vi "CLD 12 CSV file commands utility.vi"(8 "Error In":errorcluster) -> (0 "Error Out":errorcluster, 3 "Command Array Out":T1[](array[typedef]))   [LabVIEW 2019]
doc: "CLD 12: File access utility. This VI converts the text command to the enum equivalent."
uses:
  CLD 12 Data Cluster.ctl
  CLD 12 Sequencer Enum.ctl
  <vilib>/Utility/file.llb/Read Delimited Spreadsheet (string).vi
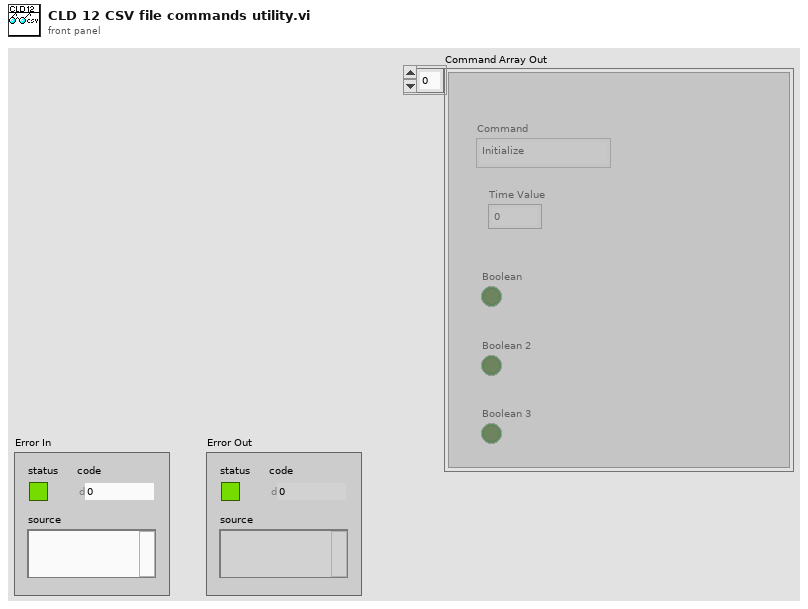
[diagram p1: front panel]
types:
  T1 = typedef "CLD 12 Data Cluster.ctl" = cluster{"Command":T2, "Time Value":dbl, "Boolean":bool, "Boolean 2":bool, "Boolean 3":bool}
  T2 = typedef "CLD 12 Sequencer Enum.ctl" = enum16{"Initialize", "SetTime", "RunState1", "Runstate2", "Idle", "Start"}
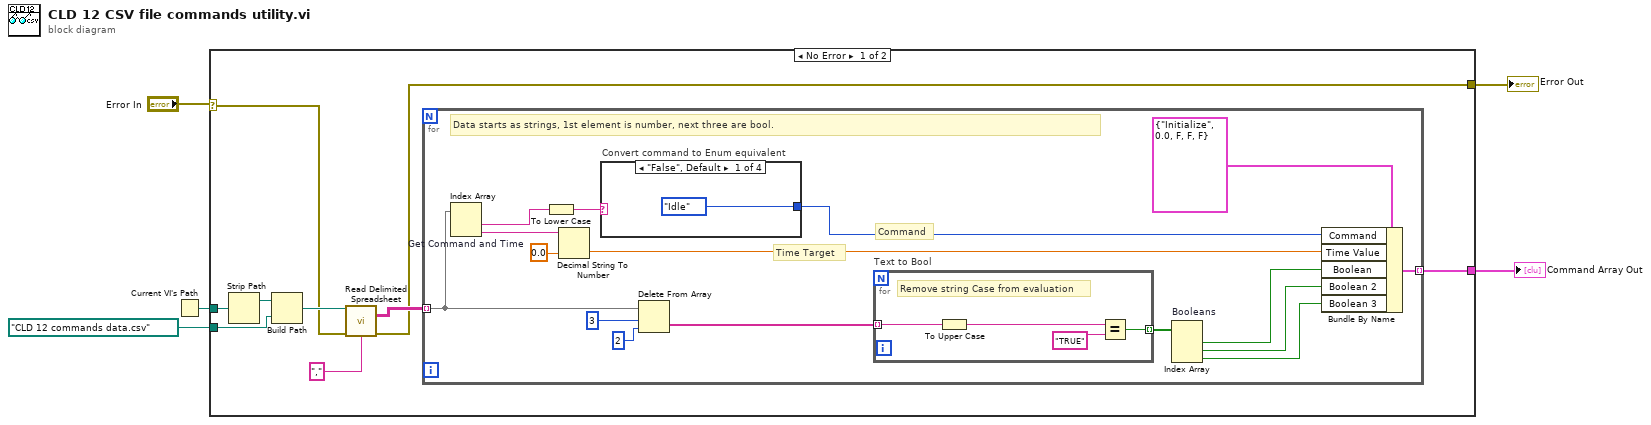
[diagram p0: block diagram]
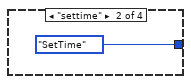
[diagram p2: hidden frame]
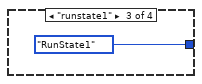
[diagram p3: hidden frame]
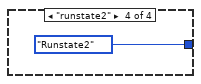
[diagram p4: hidden frame]
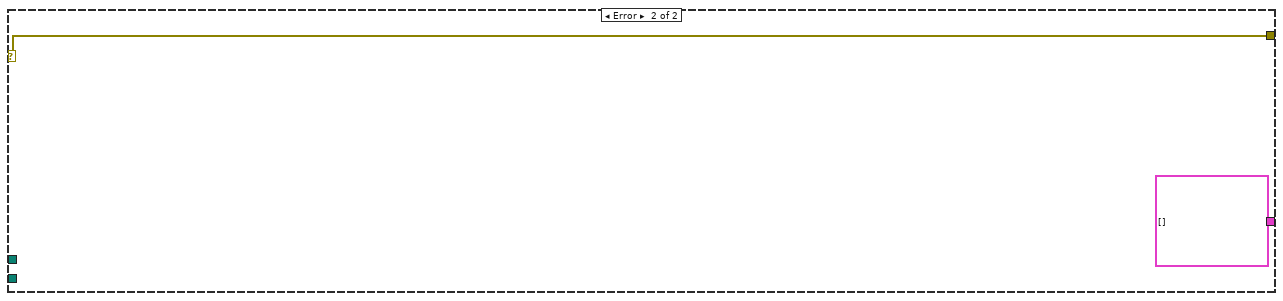
[diagram p5: hidden frame]
diagram:
  n1 = Current VI's Path() -> (path=w2:path)
  n2 = case shown="No Error" "Error In" {
    selector: "Error In" -> [w7 w40]
    tunnel: [w13 T1[] []] -> w1
    tunnel: path "CLD 12 commands data.csv" -> [w11 _]
    tunnel: w2 -> [w12 _]
    tunnel: [w6 w40] -> w3
    frame No Error {
      n3 = Strip Path(path=w12) -> (stripped path=w9:path)  [unwired: 1 out]
      n4 = Build Path(base path=w9, name or relative path=w11) -> (appended path=w10:path)
      n5 = call-poly <vilib>:"Read Delimited Spreadsheet.vi"("file path (dialog if empty)"=w10, "error in (no error)"=w7, "delimiter (\\t)"="," ("delimiter (\\t)")) -> ("all rows"=w8:string[][], "error out"=w6:errorcluster)  [unwired: 7 in, 4 out]
      n6 = for {
        tunnel: w8 -> [w30] mode=indexing
        tunnel: [w22] -> w13 mode=indexing
        # "Time Target"
        # "Command"
        # "Data starts as strings, 1st element is number, next three are bool."
        n7 = Index Array "Get Command and Time"(array=w30) -> (element #1=w18:string, element #2=w21:string)  [unwired: 2 in]
        n8 = To Lower Case(string=w18) -> (all lower case string=w16:string)
        n9 = Decimal String To Number(string=w21, default (0L)=0.0) -> (number=w20:dbl)  [unwired: 1 in, 1 out]
        n10 = case "Convert command to Enum equivalent" shown="\"False\", Default" w16 {
          tunnel: [CLD_12_Sequencer_Enum."Idle" ("Command") CLD_12_Sequencer_Enum."SetTime" ("Command") CLD_12_Sequencer_Enum."RunState1" ("Command") CLD_12_Sequencer_Enum."Runstate2" ("Command")] -> w17
          frame "False", Default {
          }
          frame "settime" {
          }
          frame "runstate1" {
          }
          frame "runstate2" {
          }
        }
        n11 = Delete From Array(array=w30, length=3, index=2) -> (deleted portion=w15:string[])  [unwired: 1 out]
        n12 = for "Text to Bool" {
          tunnel: w15 -> [w34] mode=indexing
          tunnel: [w31] -> w27 mode=indexing
          # "Remove string Case from evaluation"
          n13 = To Upper Case(1:w34) -> (0:w33:string)
          n14 = Equal?(x=w33, y="TRUE") -> (x = y?=w31:bool)
        }
        n15 = Index Array "Booleans"(array=w27) -> (element #1=w25:bool, element #2=w24:bool, element #3=w23:bool)  [unwired: 3 in]
        n16 = Bundle By Name(cluster=T1 {"Command"=enum."Initialize", "Time Value"=0.0, "Boolean"=FALSE, "Boolean 2"=FALSE, "Boolean 3"=FALSE} ("CLD 12 Data Cluster"), "Command"=w17, "Time Value"=w20, "Boolean"=w25, "Boolean 2"=w24, "Boolean 3"=w23) -> (w22:T1)
      }
    }
    frame Error {
    }
  }
  "Error Out" <- w3
  "Command Array Out" <- w1
